vi "Create 8 In Channel Resources.vi"(0 "common resources":T1={"sync pulse resources"={"sync pulse destination terminal"="", "sync100"="", "sync pulse source terminal"="", "imported sync pulse register"="", "generate sync pulse handshake"="", "enable sync pulse register"="", "sync pulse clock"=""}, "serial channel resources"={"sc 0"={"completed frames register"=""}, "sc 1"={"completed frames register"=""}, "sc 2"={"completed frames register"=""}, "sc 3"={"completed frames register"=""}, "sc 4"={"completed frames register"=""}, "sc 5"={"completed frames register"=""}, "sc 6"={"completed frames register"=""}, "sc 7"={"completed frames register"=""}}, "dram manager 0"={"DRAM class"=refnum, "process clock"="", "registers"={"configuration"={"write time slice"="", "request time slice"="", "DRAM arbiter config"="", "partition config"=""}, "reset"={"handshake"={"start.go"="", "start.go rcvd"="", "done.go"="", "done.go rcvd"=""}, "process"={"in"="", "out"=""}, "write"={"in"="", "out 0"="", "out 1"="", "out 2"="", "out 3"=""}, "read"={"in"="", "out 0"="", "out 1"="", "out 2"="", "out 3"=""}}, "status"={"partition full"=""}}, "FIFOs"={"write data"={"FIFO 0"="", "FIFO 1"="", "FIFO 2"="", "FIFO 3"=""}, "request metadata"={"FIFO"=""}, "read data VOQ"={"FIFO 0"="", "FIFO 1"="", "FIFO 2"="", "FIFO 3"=""}, "read data"={"FIFO 0"="", "FIFO 1"="", "FIFO 2"="", "FIFO 3"=""}}, "num active streams"=0.0, "max open read requests"=256}, "dram manager 1"={"DRAM class"=refnum, "process clock"="", "registers"={"configuration"={"write time slice"="", "request time slice"="", "DRAM arbiter config"="", "partition config"=""}, "reset"={"handshake"={"start.go"="", "start.go rcvd"="", "done.go"="", "done.go rcvd"=""}, "process"={"in"="", "out"=""}, "write"={"in"="", "out 0"="", "out 1"="", "out 2"="", "out 3"=""}, "read"={"in"="", "out 0"="", "out 1"="", "out 2"="", "out 3"=""}}, "status"={"partition full"=""}}, "FIFOs"={"write data"={"FIFO 0"="", "FIFO 1"="", "FIFO 2"="", "FIFO 3"=""}, "request metadata"={"FIFO"=""}, "read data VOQ"={"FIFO 0"="", "FIFO 1"="", "FIFO 2"="", "FIFO 3"=""}, "read data"={"FIFO 0"="", "FIFO 1"="", "FIFO 2"="", "FIFO 3"=""}}, "num active streams"=0.0, "max open read requests"=256}}, 5 "dram partition configs":T12[](array[typedef])=[{"first address"=0, "last address"=0}, {"first address"=0, "last address"=0}, {"first address"=0, "last address"=0}, {"first address"=0, "last address"=0}, {"first address"=0, "last address"=0}, {"first address"=0, "last address"=0}, {"first address"=0, "last address"=0}, {"first address"=0, "last address"=0}]) -> (4 "channel resources":T13)   [LabVIEW 2020, in "GettingStarted_Acq_Tap_148X_FPGA.lvlib"]
uses:
  GettingStarted_Acq_Tap_148X_FPGA.lvlib
  Types/8 In Channel Resources.ctl
  <instrlib>/_niInstr/Memory/v1/FPGA/DRAM/niInstr Memory DRAM v1 FPGA.lvclass
  Types/Serial Input Channel Resources.ctl
  <instrlib>/FlexRIO/CSI-2/v2/FPGA/DRAM Manager/Private/DRAM Manager.ctl
  <instrlib>/FlexRIO/CSI-2/v2/FPGA/DRAM Manager/Private/Common/DRAM Manager Registers.ctl
  <instrlib>/FlexRIO/CSI-2/v2/FPGA/DRAM Manager/Private/Common/Handshake Registers.ctl
  <instrlib>/FlexRIO/CSI-2/v2/FPGA/DRAM Manager/Private/Common/DRAM Manager FIFOs.ctl
  <instrlib>/FlexRIO/CSI-2/v2/FPGA/DRAM Manager/Private/Common/Write Data FIFO Ref.ctl
  <instrlib>/FlexRIO/CSI-2/v2/FPGA/DRAM Manager/Private/Common/Read Request Metadata FIFO Ref.ctl
  <instrlib>/FlexRIO/CSI-2/v2/FPGA/DRAM Manager/Private/Common/Read Data FIFO Ref.ctl
  Types/Serial Input Channel IO.ctl
  Types/Serial Input Channel IO 32b.ctl
  Types/Serial Input Channel IO 64b.ctl
  Common/Types/I2C IO.ctl
  <instrlib>/FlexRIO/CSI-2/v2/FPGA/DRAM Manager/Public/Partition Range.ctl
  Common/Types/Common Resources.ctl
  <instrlib>/FlexRIO/CSI-2/v2/FPGA/Types/Sync Pulse Resources.ctl
  Common/Types/Serial Channel Resources.ctl
  Common/Types/Single Serial Channel Resources.ctl
  <instrlib>/FlexRIO/CSI-2/v2/FPGA/DRAM Manager/DRAM Manager v2.lvlib
  Common/GettingStarted_Common_148X_FPGA.lvlib
  <instrlib>/FlexRIO/CSI-2/v2/FPGA/NI CSI-2 API FPGA v2.lvlib
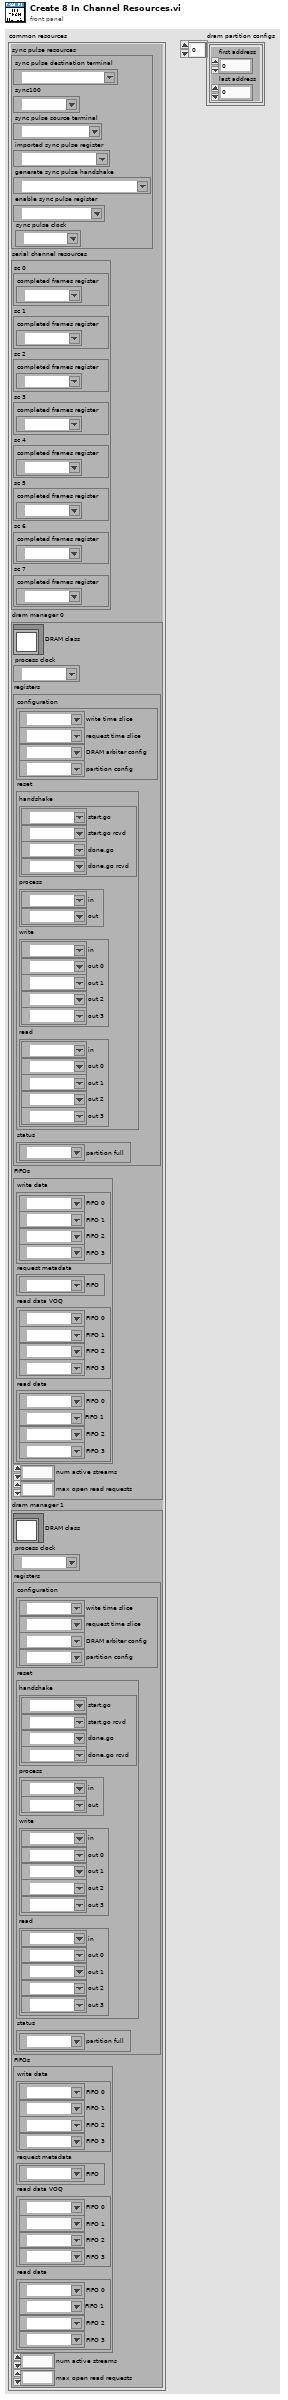
[diagram p1: front panel]
types:
  T1 = typedef "GettingStarted_Common_148X_FPGA.lvlib/Common Resources.ctl" = cluster{"sync pulse resources":T2, "serial channel resources":T3, "dram manager 0":T5, "dram manager 1":T5}
  T2 = typedef "NI CSI-2 API FPGA v2.lvlib/Sync Pulse Resources.ctl" = cluster{"sync pulse destination terminal":refnum<k21>, "sync100":refnum<k21>, "sync pulse source terminal":refnum<k21>, "imported sync pulse register":refnum<k21>, "generate sync pulse handshake":refnum<k21>, "enable sync pulse register":refnum<k21>, "sync pulse clock":refnum<k21>}
  T3 = typedef "GettingStarted_Common_148X_FPGA.lvlib/Serial Channel Resources.ctl" = cluster{"sc 0":T4, "sc 1":T4, "sc 2":T4, "sc 3":T4, "sc 4":T4, "sc 5":T4, "sc 6":T4, "sc 7":T4}
  T4 = typedef "GettingStarted_Common_148X_FPGA.lvlib/Single Serial Channel Resources.ctl" = cluster{"completed frames register":refnum<k21>}
  T5 = typedef "DRAM Manager v2.lvlib/DRAM Manager.ctl" = cluster{"DRAM class":refnum<class "niInstr Memory DRAM v1 FPGA.lvclass">, "process clock":refnum<k21>, "registers":T6, "FIFOs":T8, "num active streams":fxp<+,3,3>, "max open read requests":u16}
  T6 = typedef "DRAM Manager v2.lvlib/DRAM Manager Registers.ctl" = cluster{"configuration":cluster{"write time slice":refnum<k21>, "request time slice":refnum<k21>, "DRAM arbiter config":refnum<k21>, "partition config":refnum<k21>}, "reset":cluster{"handshake":T7, "process":cluster{"in":refnum<k21>, "out":refnum<k21>}, "write":cluster{"in":refnum<k21>, "out 0":refnum<k21>, "out 1":refnum<k21>, "out 2":refnum<k21>, "out 3":refnum<k21>}, "read":cluster{"in":refnum<k21>, "out 0":refnum<k21>, "out 1":refnum<k21>, "out 2":refnum<k21>, "out 3":refnum<k21>}}, "status":cluster{"partition full":refnum<k21>}}
  T7 = typedef "DRAM Manager v2.lvlib/Handshake Registers.ctl" = cluster{"start.go":refnum<k21>, "start.go rcvd":refnum<k21>, "done.go":refnum<k21>, "done.go rcvd":refnum<k21>}
  T8 = typedef "DRAM Manager v2.lvlib/DRAM Manager FIFOs.ctl" = cluster{"write data":cluster{"FIFO 0":T9, "FIFO 1":T9, "FIFO 2":T9, "FIFO 3":T9}, "request metadata":cluster{"FIFO":T10}, "read data VOQ":cluster{"FIFO 0":T11, "FIFO 1":T11, "FIFO 2":T11, "FIFO 3":T11}, "read data":cluster{"FIFO 0":T11, "FIFO 1":T11, "FIFO 2":T11, "FIFO 3":T11}}
  T9 = typedef "DRAM Manager v2.lvlib/Write Data FIFO Ref.ctl" = refnum<k21>
  T10 = typedef "DRAM Manager v2.lvlib/Read Request Metadata FIFO Ref.ctl" = refnum<k21>
  T11 = typedef "DRAM Manager v2.lvlib/Read Data FIFO Ref.ctl" = refnum<k21>
  T12 = typedef "DRAM Manager v2.lvlib/Partition Range.ctl" = cluster{"first address":u32, "last address":u32}
  T13 = typedef "GettingStarted_Acq_Tap_148X_FPGA.lvlib/8 In Channel Resources.ctl" = cluster{"si 0 resources":T14, "si 1 resources":T14, "si 2 resources":T14, "si 3 resources":T14, "si 4 resources":T14, "si 5 resources":T14, "si 6 resources":T14, "si 7 resources":T14}
  T14 = typedef "GettingStarted_Acq_Tap_148X_FPGA.lvlib/Serial Input Channel Resources.ctl" = cluster{"dram manager":T5, "csi-2 input io":T15, "serial input channel instance":u8, "dram stream id":fxp<+,2,2>, "i2c io":T18}
  T15 = typedef "GettingStarted_Acq_Tap_148X_FPGA.lvlib/Serial Input Channel IO.ctl" = cluster{"32b":T16, "64b":T17, "csi-2 axi stream tlast":refnum<k21>, "csi-2 axi stream tvalid":refnum<k21>}
  T16 = typedef "GettingStarted_Acq_Tap_148X_FPGA.lvlib/Serial Input Channel IO 32b.ctl" = cluster{"csi-2 axi stream tdata":refnum<k21>, "csi-2 axi stream raw tdata":refnum<k21>, "csi-2 axi stream tuser":refnum<k21>}
  T17 = typedef "GettingStarted_Acq_Tap_148X_FPGA.lvlib/Serial Input Channel IO 64b.ctl" = cluster{"csi-2 axi stream tdata":refnum<k21>, "csi-2 axi stream raw tdata":refnum<k21>, "csi-2 axi stream tuser":refnum<k21>}
  T18 = typedef "GettingStarted_Common_148X_FPGA.lvlib/I2C IO.ctl" = cluster{"sda input":refnum<k21>, "sda output enable":refnum<k21>, "scl input":refnum<k21>, "scl output enable":refnum<k21>}
  T19 = cluster{"serial input 0 csi-2 io":T15, "serial input 1 csi-2 io":T15, "serial input 2 csi-2 io":T15, "serial input 3 csi-2 io":T15, "serial input 4 csi-2 io":T15, "serial input 5 csi-2 io":T15, "serial input 6 csi-2 io":T15, "serial input 7 csi-2 io":T15}
  T20 = cluster{"serial input 0 i2c io":T18, "serial input 1 i2c io":T18, "serial input 2 i2c io":T18, "serial input 3 i2c io":T18, "serial input 4 i2c io":T18, "serial input 5 i2c io":T18, "serial input 6 i2c io":T18, "serial input 7 i2c io":T18}
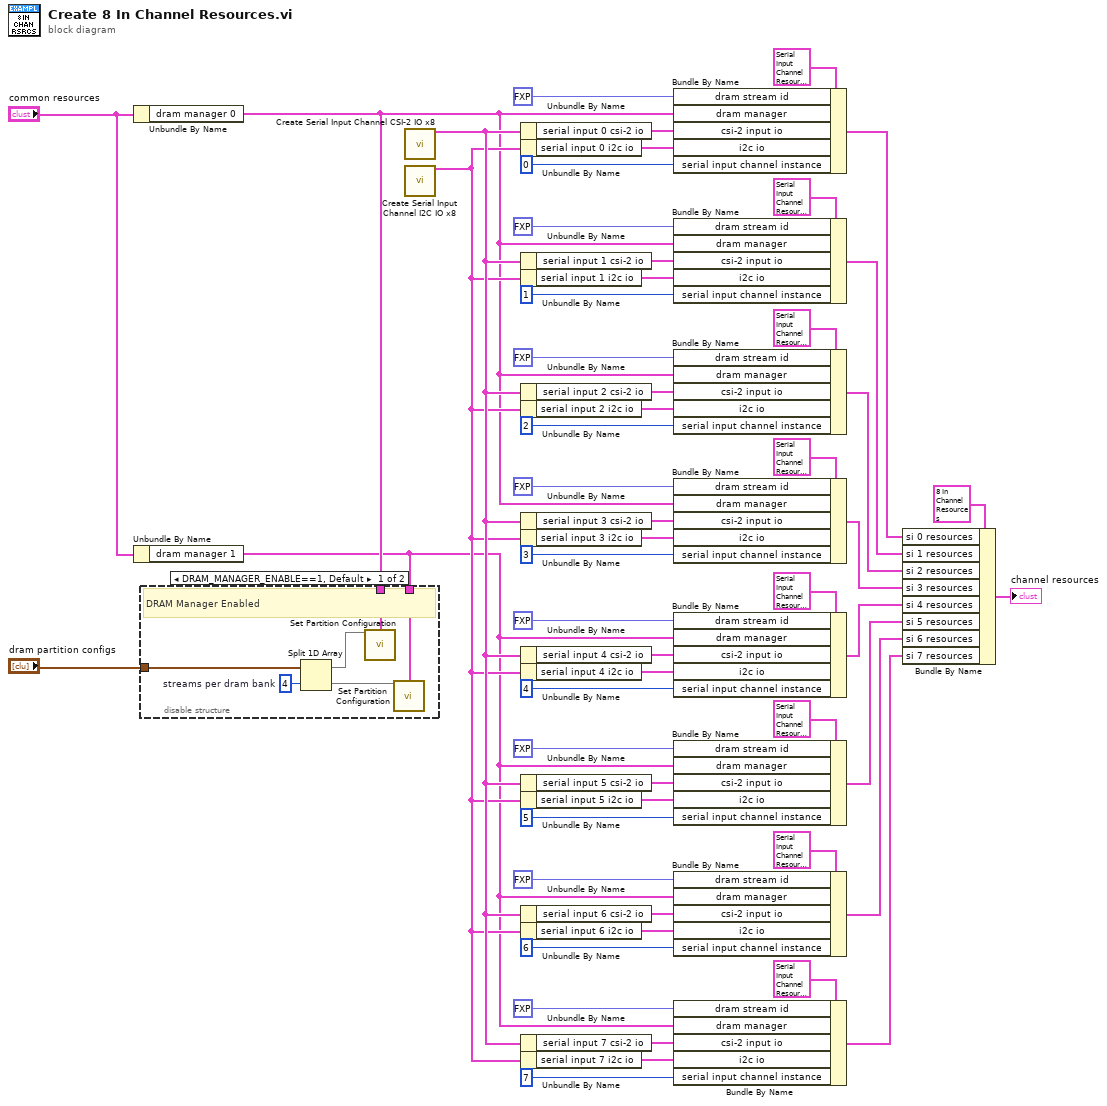
[diagram p0: block diagram]
diagram:
  n1 = Unbundle By Name("common resources") -> ("dram manager 0"=w3:T5)
  n2 = Unbundle By Name("common resources") -> ("dram manager 1"=w2:T5)
  n3 = disable-structure shown="DRAM_MANAGER_ENABLE==1, Default" {
    disable-tunnel: "dram partition configs" -> [w62 _]
    disable-tunnel: w3 -> [w58 _]
    disable-tunnel: w2 -> [w57 _]
    frame condition #0 (active) {
      w60 = 4  # streams per dram bank
      # "DRAM Manager Enabled"
      n4 = Split 1D Array(array=w62, index=w60) -> (first subarray=w61:T12[], second subarray=w59:T12[])
      n5 = call <instrlib>:"Set Partition Configuration.vi"("partition config"=w61, "DRAM manager"=w58) -> ()  [unwired: 14 in]
      n6 = call <instrlib>:"Set Partition Configuration.vi"("partition config"=w59, "DRAM manager"=w57) -> ()  [unwired: 14 in]
    }
    frame condition #1 {
      # "DRAM Manager Disabled"
    }
  }
  n7 = call "Create Serial Input Channel CSI-2 IO x8.vi"() -> ("serial input csi-2 io x8"=w5:T19)  [unwired: 15 in]
  n8 = call "Create Serial Input Channel I2C IO x8.vi"() -> ("serial input channel i2c io x8"=w4:T20)  [unwired: 15 in]
  n9 = Unbundle By Name(w5) -> ("serial input 0 csi-2 io"=w21:T15)
  n10 = Unbundle By Name(w4) -> ("serial input 0 i2c io"=w20:T18)
  n11 = Unbundle By Name(w5) -> ("serial input 1 csi-2 io"=w19:T15)
  n12 = Unbundle By Name(w4) -> ("serial input 1 i2c io"=w18:T18)
  n13 = Unbundle By Name(w5) -> ("serial input 2 csi-2 io"=w17:T15)
  n14 = Unbundle By Name(w4) -> ("serial input 2 i2c io"=w16:T18)
  n15 = Unbundle By Name(w5) -> ("serial input 3 csi-2 io"=w15:T15)
  n16 = Unbundle By Name(w4) -> ("serial input 3 i2c io"=w14:T18)
  n17 = Unbundle By Name(w5) -> ("serial input 4 csi-2 io"=w13:T15)
  n18 = Unbundle By Name(w4) -> ("serial input 4 i2c io"=w12:T18)
  n19 = Unbundle By Name(w5) -> ("serial input 5 csi-2 io"=w11:T15)
  n20 = Unbundle By Name(w4) -> ("serial input 5 i2c io"=w10:T18)
  n21 = Unbundle By Name(w5) -> ("serial input 6 csi-2 io"=w9:T15)
  n22 = Unbundle By Name(w4) -> ("serial input 6 i2c io"=w8:T18)
  n23 = Unbundle By Name(w5) -> ("serial input 7 csi-2 io"=w7:T15)
  n24 = Unbundle By Name(w4) -> ("serial input 7 i2c io"=w6:T18)
  n25 = Bundle By Name(cluster=T14 {"dram manager"={"DRAM class"=refnum, "process clock"="", "registers"={"configuration"={"write time slice"="", "request time slice"="", "DRAM arbiter config"="", "partition config"=""}, "reset"={"handshake"={"start.go"="", "start.go rcvd"="", "done.go"="", "done.go rcvd"=""}, "process"={"in"="", "out"=""}, "write"={"in"="", "out 0"="", "out 1"="", "out 2"="", "out 3"=""}, "read"={"in"="", "out 0"="", "out 1"="", "out 2"="", "out 3"=""}}, "status"={"partition full"=""}}, "FIFOs"={"write data"={"FIFO 0"="", "FIFO 1"="", "FIFO 2"="", "FIFO 3"=""}, "request metadata"={"FIFO"=""}, "read data VOQ"={"FIFO 0"="", "FIFO 1"="", "FIFO 2"="", "FIFO 3"=""}, "read data"={"FIFO 0"="", "FIFO 1"="", "FIFO 2"="", "FIFO 3"=""}}, "num active streams"=0.0, "max open read requests"=0}, "csi-2 input io"={"32b"={"csi-2 axi stream tdata"="", "csi-2 axi stream raw tdata"="", "csi-2 axi stream tuser"=""}, "64b"={"csi-2 axi stream tdata"="", "csi-2 axi stream raw tdata"="", "csi-2 axi stream tuser"=""}, "csi-2 axi stream tlast"="", "csi-2 axi stream tvalid"=""}, "serial input channel instance"=0, "dram stream id"=0.0, "i2c io"={"sda input"="", "sda output enable"="", "scl input"="", "scl output enable"=""}} ("si 0 resources"), "dram stream id"=fxp<+,2,2> 0.0, "dram manager"=w3, "csi-2 input io"=w21, "i2c io"=w20, "serial input channel instance"=u8 0) -> (w51:T14)
  n26 = Bundle By Name(cluster=T14 {"dram manager"={"DRAM class"=refnum, "process clock"="", "registers"={"configuration"={"write time slice"="", "request time slice"="", "DRAM arbiter config"="", "partition config"=""}, "reset"={"handshake"={"start.go"="", "start.go rcvd"="", "done.go"="", "done.go rcvd"=""}, "process"={"in"="", "out"=""}, "write"={"in"="", "out 0"="", "out 1"="", "out 2"="", "out 3"=""}, "read"={"in"="", "out 0"="", "out 1"="", "out 2"="", "out 3"=""}}, "status"={"partition full"=""}}, "FIFOs"={"write data"={"FIFO 0"="", "FIFO 1"="", "FIFO 2"="", "FIFO 3"=""}, "request metadata"={"FIFO"=""}, "read data VOQ"={"FIFO 0"="", "FIFO 1"="", "FIFO 2"="", "FIFO 3"=""}, "read data"={"FIFO 0"="", "FIFO 1"="", "FIFO 2"="", "FIFO 3"=""}}, "num active streams"=0.0, "max open read requests"=0}, "csi-2 input io"={"32b"={"csi-2 axi stream tdata"="", "csi-2 axi stream raw tdata"="", "csi-2 axi stream tuser"=""}, "64b"={"csi-2 axi stream tdata"="", "csi-2 axi stream raw tdata"="", "csi-2 axi stream tuser"=""}, "csi-2 axi stream tlast"="", "csi-2 axi stream tvalid"=""}, "serial input channel instance"=0, "dram stream id"=0.0, "i2c io"={"sda input"="", "sda output enable"="", "scl input"="", "scl output enable"=""}} ("si 0 resources"), "dram stream id"=fxp<+,2,2> 1.0, "dram manager"=w3, "csi-2 input io"=w19, "i2c io"=w18, "serial input channel instance"=u8 1) -> (w47:T14)
  n27 = Bundle By Name(cluster=T14 {"dram manager"={"DRAM class"=refnum, "process clock"="", "registers"={"configuration"={"write time slice"="", "request time slice"="", "DRAM arbiter config"="", "partition config"=""}, "reset"={"handshake"={"start.go"="", "start.go rcvd"="", "done.go"="", "done.go rcvd"=""}, "process"={"in"="", "out"=""}, "write"={"in"="", "out 0"="", "out 1"="", "out 2"="", "out 3"=""}, "read"={"in"="", "out 0"="", "out 1"="", "out 2"="", "out 3"=""}}, "status"={"partition full"=""}}, "FIFOs"={"write data"={"FIFO 0"="", "FIFO 1"="", "FIFO 2"="", "FIFO 3"=""}, "request metadata"={"FIFO"=""}, "read data VOQ"={"FIFO 0"="", "FIFO 1"="", "FIFO 2"="", "FIFO 3"=""}, "read data"={"FIFO 0"="", "FIFO 1"="", "FIFO 2"="", "FIFO 3"=""}}, "num active streams"=0.0, "max open read requests"=0}, "csi-2 input io"={"32b"={"csi-2 axi stream tdata"="", "csi-2 axi stream raw tdata"="", "csi-2 axi stream tuser"=""}, "64b"={"csi-2 axi stream tdata"="", "csi-2 axi stream raw tdata"="", "csi-2 axi stream tuser"=""}, "csi-2 axi stream tlast"="", "csi-2 axi stream tvalid"=""}, "serial input channel instance"=0, "dram stream id"=0.0, "i2c io"={"sda input"="", "sda output enable"="", "scl input"="", "scl output enable"=""}} ("si 0 resources"), "dram stream id"=fxp<+,2,2> 2.0, "dram manager"=w3, "csi-2 input io"=w17, "i2c io"=w16, "serial input channel instance"=u8 2) -> (w43:T14)
  n28 = Bundle By Name(cluster=T14 {"dram manager"={"DRAM class"=refnum, "process clock"="", "registers"={"configuration"={"write time slice"="", "request time slice"="", "DRAM arbiter config"="", "partition config"=""}, "reset"={"handshake"={"start.go"="", "start.go rcvd"="", "done.go"="", "done.go rcvd"=""}, "process"={"in"="", "out"=""}, "write"={"in"="", "out 0"="", "out 1"="", "out 2"="", "out 3"=""}, "read"={"in"="", "out 0"="", "out 1"="", "out 2"="", "out 3"=""}}, "status"={"partition full"=""}}, "FIFOs"={"write data"={"FIFO 0"="", "FIFO 1"="", "FIFO 2"="", "FIFO 3"=""}, "request metadata"={"FIFO"=""}, "read data VOQ"={"FIFO 0"="", "FIFO 1"="", "FIFO 2"="", "FIFO 3"=""}, "read data"={"FIFO 0"="", "FIFO 1"="", "FIFO 2"="", "FIFO 3"=""}}, "num active streams"=0.0, "max open read requests"=0}, "csi-2 input io"={"32b"={"csi-2 axi stream tdata"="", "csi-2 axi stream raw tdata"="", "csi-2 axi stream tuser"=""}, "64b"={"csi-2 axi stream tdata"="", "csi-2 axi stream raw tdata"="", "csi-2 axi stream tuser"=""}, "csi-2 axi stream tlast"="", "csi-2 axi stream tvalid"=""}, "serial input channel instance"=0, "dram stream id"=0.0, "i2c io"={"sda input"="", "sda output enable"="", "scl input"="", "scl output enable"=""}} ("si 0 resources"), "dram stream id"=fxp<+,2,2> 3.0, "dram manager"=w3, "csi-2 input io"=w15, "i2c io"=w14, "serial input channel instance"=u8 3) -> (w39:T14)
  n29 = Bundle By Name(cluster=T14 {"dram manager"={"DRAM class"=refnum, "process clock"="", "registers"={"configuration"={"write time slice"="", "request time slice"="", "DRAM arbiter config"="", "partition config"=""}, "reset"={"handshake"={"start.go"="", "start.go rcvd"="", "done.go"="", "done.go rcvd"=""}, "process"={"in"="", "out"=""}, "write"={"in"="", "out 0"="", "out 1"="", "out 2"="", "out 3"=""}, "read"={"in"="", "out 0"="", "out 1"="", "out 2"="", "out 3"=""}}, "status"={"partition full"=""}}, "FIFOs"={"write data"={"FIFO 0"="", "FIFO 1"="", "FIFO 2"="", "FIFO 3"=""}, "request metadata"={"FIFO"=""}, "read data VOQ"={"FIFO 0"="", "FIFO 1"="", "FIFO 2"="", "FIFO 3"=""}, "read data"={"FIFO 0"="", "FIFO 1"="", "FIFO 2"="", "FIFO 3"=""}}, "num active streams"=0.0, "max open read requests"=0}, "csi-2 input io"={"32b"={"csi-2 axi stream tdata"="", "csi-2 axi stream raw tdata"="", "csi-2 axi stream tuser"=""}, "64b"={"csi-2 axi stream tdata"="", "csi-2 axi stream raw tdata"="", "csi-2 axi stream tuser"=""}, "csi-2 axi stream tlast"="", "csi-2 axi stream tvalid"=""}, "serial input channel instance"=0, "dram stream id"=0.0, "i2c io"={"sda input"="", "sda output enable"="", "scl input"="", "scl output enable"=""}} ("si 0 resources"), "dram stream id"=fxp<+,2,2> 0.0, "dram manager"=w2, "csi-2 input io"=w13, "i2c io"=w12, "serial input channel instance"=u8 4) -> (w35:T14)
  n30 = Bundle By Name(cluster=T14 {"dram manager"={"DRAM class"=refnum, "process clock"="", "registers"={"configuration"={"write time slice"="", "request time slice"="", "DRAM arbiter config"="", "partition config"=""}, "reset"={"handshake"={"start.go"="", "start.go rcvd"="", "done.go"="", "done.go rcvd"=""}, "process"={"in"="", "out"=""}, "write"={"in"="", "out 0"="", "out 1"="", "out 2"="", "out 3"=""}, "read"={"in"="", "out 0"="", "out 1"="", "out 2"="", "out 3"=""}}, "status"={"partition full"=""}}, "FIFOs"={"write data"={"FIFO 0"="", "FIFO 1"="", "FIFO 2"="", "FIFO 3"=""}, "request metadata"={"FIFO"=""}, "read data VOQ"={"FIFO 0"="", "FIFO 1"="", "FIFO 2"="", "FIFO 3"=""}, "read data"={"FIFO 0"="", "FIFO 1"="", "FIFO 2"="", "FIFO 3"=""}}, "num active streams"=0.0, "max open read requests"=0}, "csi-2 input io"={"32b"={"csi-2 axi stream tdata"="", "csi-2 axi stream raw tdata"="", "csi-2 axi stream tuser"=""}, "64b"={"csi-2 axi stream tdata"="", "csi-2 axi stream raw tdata"="", "csi-2 axi stream tuser"=""}, "csi-2 axi stream tlast"="", "csi-2 axi stream tvalid"=""}, "serial input channel instance"=0, "dram stream id"=0.0, "i2c io"={"sda input"="", "sda output enable"="", "scl input"="", "scl output enable"=""}} ("si 0 resources"), "dram stream id"=fxp<+,2,2> 1.0, "dram manager"=w2, "csi-2 input io"=w11, "i2c io"=w10, "serial input channel instance"=u8 5) -> (w31:T14)
  n31 = Bundle By Name(cluster=T14 {"dram manager"={"DRAM class"=refnum, "process clock"="", "registers"={"configuration"={"write time slice"="", "request time slice"="", "DRAM arbiter config"="", "partition config"=""}, "reset"={"handshake"={"start.go"="", "start.go rcvd"="", "done.go"="", "done.go rcvd"=""}, "process"={"in"="", "out"=""}, "write"={"in"="", "out 0"="", "out 1"="", "out 2"="", "out 3"=""}, "read"={"in"="", "out 0"="", "out 1"="", "out 2"="", "out 3"=""}}, "status"={"partition full"=""}}, "FIFOs"={"write data"={"FIFO 0"="", "FIFO 1"="", "FIFO 2"="", "FIFO 3"=""}, "request metadata"={"FIFO"=""}, "read data VOQ"={"FIFO 0"="", "FIFO 1"="", "FIFO 2"="", "FIFO 3"=""}, "read data"={"FIFO 0"="", "FIFO 1"="", "FIFO 2"="", "FIFO 3"=""}}, "num active streams"=0.0, "max open read requests"=0}, "csi-2 input io"={"32b"={"csi-2 axi stream tdata"="", "csi-2 axi stream raw tdata"="", "csi-2 axi stream tuser"=""}, "64b"={"csi-2 axi stream tdata"="", "csi-2 axi stream raw tdata"="", "csi-2 axi stream tuser"=""}, "csi-2 axi stream tlast"="", "csi-2 axi stream tvalid"=""}, "serial input channel instance"=0, "dram stream id"=0.0, "i2c io"={"sda input"="", "sda output enable"="", "scl input"="", "scl output enable"=""}} ("si 0 resources"), "dram stream id"=fxp<+,2,2> 2.0, "dram manager"=w2, "csi-2 input io"=w9, "i2c io"=w8, "serial input channel instance"=u8 6) -> (w27:T14)
  n32 = Bundle By Name(cluster=T14 {"dram manager"={"DRAM class"=refnum, "process clock"="", "registers"={"configuration"={"write time slice"="", "request time slice"="", "DRAM arbiter config"="", "partition config"=""}, "reset"={"handshake"={"start.go"="", "start.go rcvd"="", "done.go"="", "done.go rcvd"=""}, "process"={"in"="", "out"=""}, "write"={"in"="", "out 0"="", "out 1"="", "out 2"="", "out 3"=""}, "read"={"in"="", "out 0"="", "out 1"="", "out 2"="", "out 3"=""}}, "status"={"partition full"=""}}, "FIFOs"={"write data"={"FIFO 0"="", "FIFO 1"="", "FIFO 2"="", "FIFO 3"=""}, "request metadata"={"FIFO"=""}, "read data VOQ"={"FIFO 0"="", "FIFO 1"="", "FIFO 2"="", "FIFO 3"=""}, "read data"={"FIFO 0"="", "FIFO 1"="", "FIFO 2"="", "FIFO 3"=""}}, "num active streams"=0.0, "max open read requests"=0}, "csi-2 input io"={"32b"={"csi-2 axi stream tdata"="", "csi-2 axi stream raw tdata"="", "csi-2 axi stream tuser"=""}, "64b"={"csi-2 axi stream tdata"="", "csi-2 axi stream raw tdata"="", "csi-2 axi stream tuser"=""}, "csi-2 axi stream tlast"="", "csi-2 axi stream tvalid"=""}, "serial input channel instance"=0, "dram stream id"=0.0, "i2c io"={"sda input"="", "sda output enable"="", "scl input"="", "scl output enable"=""}} ("si 0 resources"), "dram stream id"=fxp<+,2,2> 3.0, "dram manager"=w2, "csi-2 input io"=w7, "i2c io"=w6, "serial input channel instance"=u8 7) -> (w23:T14)
  n33 = Bundle By Name(cluster=T13 {"si 0 resources"={"dram manager"={"DRAM class"=refnum, "process clock"="", "registers"={"configuration"={"write time slice"="", "request time slice"="", "DRAM arbiter config"="", "partition config"=""}, "reset"={"handshake"={"start.go"="", "start.go rcvd"="", "done.go"="", "done.go rcvd"=""}, "process"={"in"="", "out"=""}, "write"={"in"="", "out 0"="", "out 1"="", "out 2"="", "out 3"=""}, "read"={"in"="", "out 0"="", "out 1"="", "out 2"="", "out 3"=""}}, "status"={"partition full"=""}}, "FIFOs"={"write data"={"FIFO 0"="", "FIFO 1"="", "FIFO 2"="", "FIFO 3"=""}, "request metadata"={"FIFO"=""}, "read data VOQ"={"FIFO 0"="", "FIFO 1"="", "FIFO 2"="", "FIFO 3"=""}, "read data"={"FIFO 0"="", "FIFO 1"="", "FIFO 2"="", "FIFO 3"=""}}, "num active streams"=0.0, "max open read requests"=0}, "csi-2 input io"={"32b"={"csi-2 axi stream tdata"="", "csi-2 axi stream raw tdata"="", "csi-2 axi stream tuser"=""}, "64b"={"csi-2 axi stream tdata"="", "csi-2 axi stream raw tdata"="", "csi-2 axi stream tuser"=""}, "csi-2 axi stream tlast"="", "csi-2 axi stream tvalid"=""}, "serial input channel instance"=0, "dram stream id"=0.0, "i2c io"={"sda input"="", "sda output enable"="", "scl input"="", "scl output enable"=""}}, "si 1 resources"={"dram manager"={"DRAM class"=refnum, "process clock"="", "registers"={"configuration"={"write time slice"="", "request time slice"="", "DRAM arbiter config"="", "partition config"=""}, "reset"={"handshake"={"start.go"="", "start.go rcvd"="", "done.go"="", "done.go rcvd"=""}, "process"={"in"="", "out"=""}, "write"={"in"="", "out 0"="", "out 1"="", "out 2"="", "out 3"=""}, "read"={"in"="", "out 0"="", "out 1"="", "out 2"="", "out 3"=""}}, "status"={"partition full"=""}}, "FIFOs"={"write data"={"FIFO 0"="", "FIFO 1"="", "FIFO 2"="", "FIFO 3"=""}, "request metadata"={"FIFO"=""}, "read data VOQ"={"FIFO 0"="", "FIFO 1"="", "FIFO 2"="", "FIFO 3"=""}, "read data"={"FIFO 0"="", "FIFO 1"="", "FIFO 2"="", "FIFO 3"=""}}, "num active streams"=0.0, "max open read requests"=0}, "csi-2 input io"={"32b"={"csi-2 axi stream tdata"="", "csi-2 axi stream raw tdata"="", "csi-2 axi stream tuser"=""}, "64b"={"csi-2 axi stream tdata"="", "csi-2 axi stream raw tdata"="", "csi-2 axi stream tuser"=""}, "csi-2 axi stream tlast"="", "csi-2 axi stream tvalid"=""}, "serial input channel instance"=0, "dram stream id"=0.0, "i2c io"={"sda input"="", "sda output enable"="", "scl input"="", "scl output enable"=""}}, "si 2 resources"={"dram manager"={"DRAM class"=refnum, "process clock"="", "registers"={"configuration"={"write time slice"="", "request time slice"="", "DRAM arbiter config"="", "partition config"=""}, "reset"={"handshake"={"start.go"="", "start.go rcvd"="", "done.go"="", "done.go rcvd"=""}, "process"={"in"="", "out"=""}, "write"={"in"="", "out 0"="", "out 1"="", "out 2"="", "out 3"=""}, "read"={"in"="", "out 0"="", "out 1"="", "out 2"="", "out 3"=""}}, "status"={"partition full"=""}}, "FIFOs"={"write data"={"FIFO 0"="", "FIFO 1"="", "FIFO 2"="", "FIFO 3"=""}, "request metadata"={"FIFO"=""}, "read data VOQ"={"FIFO 0"="", "FIFO 1"="", "FIFO 2"="", "FIFO 3"=""}, "read data"={"FIFO 0"="", "FIFO 1"="", "FIFO 2"="", "FIFO 3"=""}}, "num active streams"=0.0, "max open read requests"=0}, "csi-2 input io"={"32b"={"csi-2 axi stream tdata"="", "csi-2 axi stream raw tdata"="", "csi-2 axi stream tuser"=""}, "64b"={"csi-2 axi stream tdata"="", "csi-2 axi stream raw tdata"="", "csi-2 axi stream tuser"=""}, "csi-2 axi stream tlast"="", "csi-2 axi stream tvalid"=""}, "serial input channel instance"=0, "dram stream id"=0.0, "i2c io"={"sda input"="", "sda output enable"="", "scl input"="", "scl output enable"=""}}, "si 3 resources"={"dram manager"={"DRAM class"=refnum, "process clock"="", "registers"={"configuration"={"write time slice"="", "request time slice"="", "DRAM arbiter config"="", "partition config"=""}, "reset"={"handshake"={"start.go"="", "start.go rcvd"="", "done.go"="", "done.go rcvd"=""}, "process"={"in"="", "out"=""}, "write"={"in"="", "out 0"="", "out 1"="", "out 2"="", "out 3"=""}, "read"={"in"="", "out 0"="", "out 1"="", "out 2"="", "out 3"=""}}, "status"={"partition full"=""}}, "FIFOs"={"write data"={"FIFO 0"="", "FIFO 1"="", "FIFO 2"="", "FIFO 3"=""}, "request metadata"={"FIFO"=""}, "read data VOQ"={"FIFO 0"="", "FIFO 1"="", "FIFO 2"="", "FIFO 3"=""}, "read data"={"FIFO 0"="", "FIFO 1"="", "FIFO 2"="", "FIFO 3"=""}}, "num active streams"=0.0, "max open read requests"=0}, "csi-2 input io"={"32b"={"csi-2 axi stream tdata"="", "csi-2 axi stream raw tdata"="", "csi-2 axi stream tuser"=""}, "64b"={"csi-2 axi stream tdata"="", "csi-2 axi stream raw tdata"="", "csi-2 axi stream tuser"=""}, "csi-2 axi stream tlast"="", "csi-2 axi stream tvalid"=""}, "serial input channel instance"=0, "dram stream id"=0.0, "i2c io"={"sda input"="", "sda output enable"="", "scl input"="", "scl output enable"=""}}, "si 4 resources"={"dram manager"={"DRAM class"=refnum, "process clock"="", "registers"={"configuration"={"write time slice"="", "request time slice"="", "DRAM arbiter config"="", "partition config"=""}, "reset"={"handshake"={"start.go"="", "start.go rcvd"="", "done.go"="", "done.go rcvd"=""}, "process"={"in"="", "out"=""}, "write"={"in"="", "out 0"="", "out 1"="", "out 2"="", "out 3"=""}, "read"={"in"="", "out 0"="", "out 1"="", "out 2"="", "out 3"=""}}, "status"={"partition full"=""}}, "FIFOs"={"write data"={"FIFO 0"="", "FIFO 1"="", "FIFO 2"="", "FIFO 3"=""}, "request metadata"={"FIFO"=""}, "read data VOQ"={"FIFO 0"="", "FIFO 1"="", "FIFO 2"="", "FIFO 3"=""}, "read data"={"FIFO 0"="", "FIFO 1"="", "FIFO 2"="", "FIFO 3"=""}}, "num active streams"=0.0, "max open read requests"=0}, "csi-2 input io"={"32b"={"csi-2 axi stream tdata"="", "csi-2 axi stream raw tdata"="", "csi-2 axi stream tuser"=""}, "64b"={"csi-2 axi stream tdata"="", "csi-2 axi stream raw tdata"="", "csi-2 axi stream tuser"=""}, "csi-2 axi stream tlast"="", "csi-2 axi stream tvalid"=""}, "serial input channel instance"=0, "dram stream id"=0.0, "i2c io"={"sda input"="", "sda output enable"="", "scl input"="", "scl output enable"=""}}, "si 5 resources"={"dram manager"={"DRAM class"=refnum, "process clock"="", "registers"={"configuration"={"write time slice"="", "request time slice"="", "DRAM arbiter config"="", "partition config"=""}, "reset"={"handshake"={"start.go"="", "start.go rcvd"="", "done.go"="", "done.go rcvd"=""}, "process"={"in"="", "out"=""}, "write"={"in"="", "out 0"="", "out 1"="", "out 2"="", "out 3"=""}, "read"={"in"="", "out 0"="", "out 1"="", "out 2"="", "out 3"=""}}, "status"={"partition full"=""}}, "FIFOs"={"write data"={"FIFO 0"="", "FIFO 1"="", "FIFO 2"="", "FIFO 3"=""}, "request metadata"={"FIFO"=""}, "read data VOQ"={"FIFO 0"="", "FIFO 1"="", "FIFO 2"="", "FIFO 3"=""}, "read data"={"FIFO 0"="", "FIFO 1"="", "FIFO 2"="", "FIFO 3"=""}}, "num active streams"=0.0, "max open read requests"=0}, "csi-2 input io"={"32b"={"csi-2 axi stream tdata"="", "csi-2 axi stream raw tdata"="", "csi-2 axi stream tuser"=""}, "64b"={"csi-2 axi stream tdata"="", "csi-2 axi stream raw tdata"="", "csi-2 axi stream tuser"=""}, "csi-2 axi stream tlast"="", "csi-2 axi stream tvalid"=""}, "serial input channel instance"=0, "dram stream id"=0.0, "i2c io"={"sda input"="", "sda output enable"="", "scl input"="", "scl output enable"=""}}, "si 6 resources"={"dram manager"={"DRAM class"=refnum, "process clock"="", "registers"={"configuration"={"write time slice"="", "request time slice"="", "DRAM arbiter config"="", "partition config"=""}, "reset"={"handshake"={"start.go"="", "start.go rcvd"="", "done.go"="", "done.go rcvd"=""}, "process"={"in"="", "out"=""}, "write"={"in"="", "out 0"="", "out 1"="", "out 2"="", "out 3"=""}, "read"={"in"="", "out 0"="", "out 1"="", "out 2"="", "out 3"=""}}, "status"={"partition full"=""}}, "FIFOs"={"write data"={"FIFO 0"="", "FIFO 1"="", "FIFO 2"="", "FIFO 3"=""}, "request metadata"={"FIFO"=""}, "read data VOQ"={"FIFO 0"="", "FIFO 1"="", "FIFO 2"="", "FIFO 3"=""}, "read data"={"FIFO 0"="", "FIFO 1"="", "FIFO 2"="", "FIFO 3"=""}}, "num active streams"=0.0, "max open read requests"=0}, "csi-2 input io"={"32b"={"csi-2 axi stream tdata"="", "csi-2 axi stream raw tdata"="", "csi-2 axi stream tuser"=""}, "64b"={"csi-2 axi stream tdata"="", "csi-2 axi stream raw tdata"="", "csi-2 axi stream tuser"=""}, "csi-2 axi stream tlast"="", "csi-2 axi stream tvalid"=""}, "serial input channel instance"=0, "dram stream id"=0.0, "i2c io"={"sda input"="", "sda output enable"="", "scl input"="", "scl output enable"=""}}, "si 7 resources"={"dram manager"={"DRAM class"=refnum, "process clock"="", "registers"={"configuration"={"write time slice"="", "request time slice"="", "DRAM arbiter config"="", "partition config"=""}, "reset"={"handshake"={"start.go"="", "start.go rcvd"="", "done.go"="", "done.go rcvd"=""}, "process"={"in"="", "out"=""}, "write"={"in"="", "out 0"="", "out 1"="", "out 2"="", "out 3"=""}, "read"={"in"="", "out 0"="", "out 1"="", "out 2"="", "out 3"=""}}, "status"={"partition full"=""}}, "FIFOs"={"write data"={"FIFO 0"="", "FIFO 1"="", "FIFO 2"="", "FIFO 3"=""}, "request metadata"={"FIFO"=""}, "read data VOQ"={"FIFO 0"="", "FIFO 1"="", "FIFO 2"="", "FIFO 3"=""}, "read data"={"FIFO 0"="", "FIFO 1"="", "FIFO 2"="", "FIFO 3"=""}}, "num active streams"=0.0, "max open read requests"=0}, "csi-2 input io"={"32b"={"csi-2 axi stream tdata"="", "csi-2 axi stream raw tdata"="", "csi-2 axi stream tuser"=""}, "64b"={"csi-2 axi stream tdata"="", "csi-2 axi stream raw tdata"="", "csi-2 axi stream tuser"=""}, "csi-2 axi stream tlast"="", "csi-2 axi stream tvalid"=""}, "serial input channel instance"=0, "dram stream id"=0.0, "i2c io"={"sda input"="", "sda output enable"="", "scl input"="", "scl output enable"=""}}} ("8 In Channel Resources"), "si 0 resources"=w51, "si 1 resources"=w47, "si 2 resources"=w43, "si 3 resources"=w39, "si 4 resources"=w35, "si 5 resources"=w31, "si 6 resources"=w27, "si 7 resources"=w23) -> (→"channel resources":T13)
